vi "Task_03.vi"() -> ()   [LabVIEW 2018]
uses:
  Histogram.ctl
  Stat_cluster.ctl
  <vilib>/Utility/file.llb/Write Delimited Spreadsheet (DBL).vi
panel:
  out "File write error":errorcluster
  out "Histogramm 2":T1
  out "Stats 2":T2
  out "Stats":T2
  out "Histogramm":T1
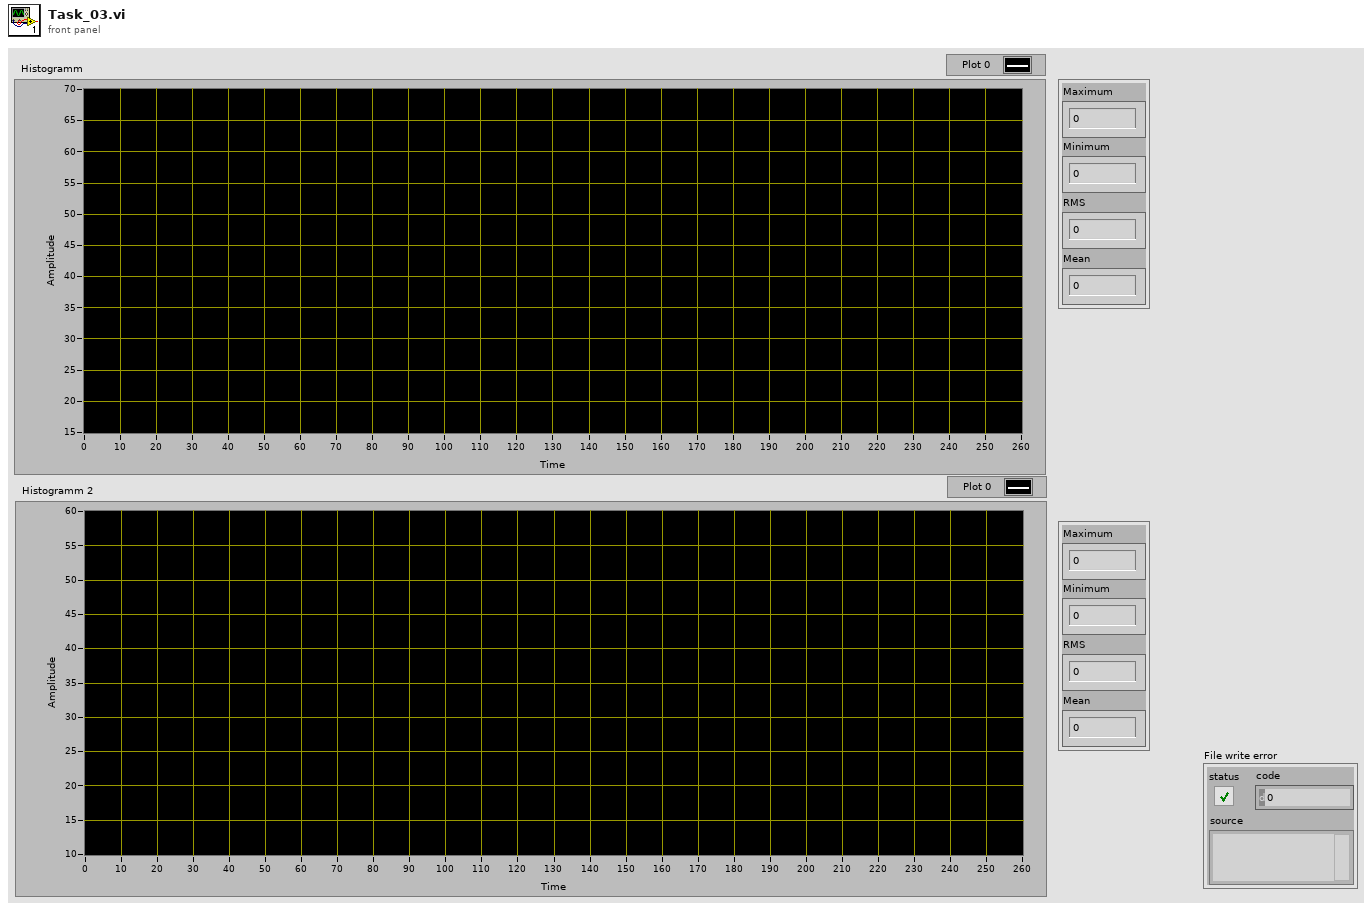
[diagram p1: front panel]
types:
  T1 = typedef "Histogram.ctl" = cluster{"X Values":dbl[], "Histogram: h(x)":i32[]}
  T2 = typedef "Stat_cluster.ctl" = cluster{"Maximum":dbl, "Minimum":dbl, "RMS":dbl, "Mean":dbl}
  T3 = cluster{"Numeric Control":u8, "Numeric Control":u8, "rms value":dbl, "mean":dbl}
  T4 = cluster{"X Values":dbl[], "Histogram: h(x)":i32[]}
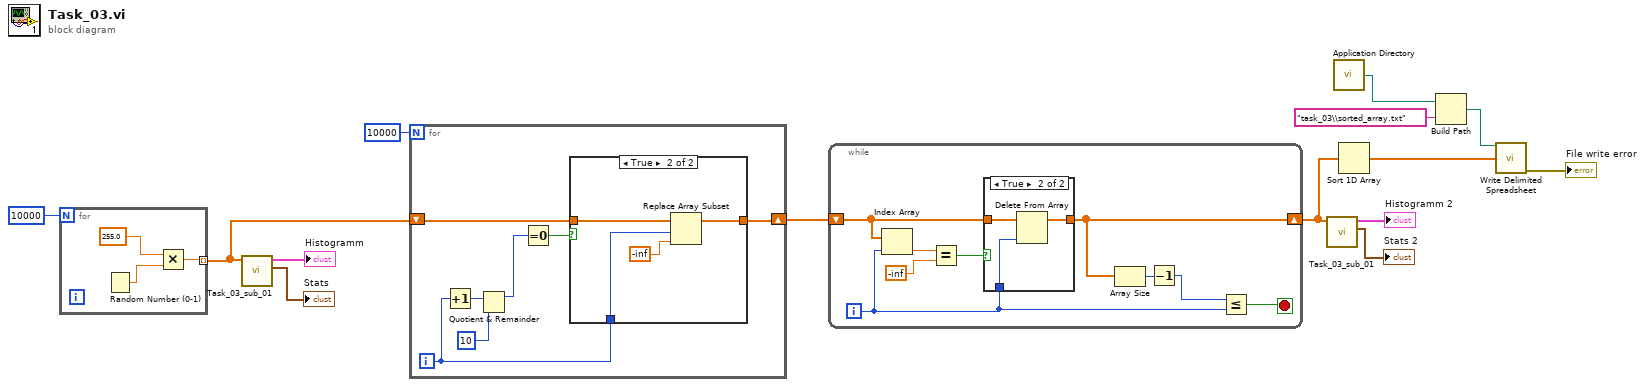
[diagram p0: block diagram]
diagram:
  n1 = for {
    N: 10000 -> [_]
    tunnel: [w15] -> w10 mode=indexing
    n2 = Random Number (0-1)() -> (number: 0 to 1=w16:dbl)
    n3 = Multiply(x=255.0, y=w16) -> (x*y=w15:dbl)
  }
  n4 = call "Task_03_sub_01.vi"("Array"=w10) -> ("Stat_Cluster"=→"Stats":T3, "Histogram Graph"=→"Histogramm":T4)  [unwired: 9 in]
  n5 = for {
    N: 10000 -> [_]
    shift-right: [w19] -> w9
    shift-left: w10 -> [w20]
    i -> [w21]
    n6 = Increment(x=w21) -> (x+1=w24:i32)
    n7 = Quotient & Remainder(x=w24, y=10) -> (x-y*floor(x/y)=w18:i32)  [unwired: 1 out]
    n8 = Equal To 0?(x=w18) -> (x = 0?=w22:bool)
    n9 = case shown="True" w22 {
      tunnel: w21 -> [_ w28]
      tunnel: w20 -> [w25 w29]
      tunnel: [w25 w27] -> w19
      frame False {
      }
      frame True {
        n10 = Replace Array Subset(array=w29, new element=-inf, index=w28) -> (w27:dbl[])
      }
    }
  }
  n11 = while {
    shift-right: [w35] -> w6
    shift-left: w9 -> [w37]
    i -> [w32]
    stop <- w31 stop-if-true
    n12 = Index Array(array=w37, index=w32) -> (element=w38:dbl)
    n13 = Equal?(x=w38, y=-inf) -> (x = y?=w36:bool)
    n14 = case shown="True" w36 {
      tunnel: w37 -> [w39 w42]
      tunnel: w32 -> [_ w41]
      tunnel: [w39 w40] -> w35
      frame False {
      }
      frame True {
        n15 = Delete From Array(array=w42, index=w41) -> (array with subset deleted=w40:dbl[])  [unwired: 1 in, 1 out]
      }
    }
    n16 = Array Size(array=w35) -> (size(s)=w34:i32)
    n17 = Decrement(x=w34) -> (x-1=w33:i32)
    n18 = Less Or Equal?(x=w33, y=w32) -> (x <= y?=w31:bool)
  }
  n19 = call "Task_03_sub_01.vi"("Array"=w6) -> ("Stat_Cluster"=→"Stats 2":T3, "Histogram Graph"=→"Histogramm 2":T4)  [unwired: 9 in]
  n20 = call <vilib>:"Application Directory.vi"() -> ("Application Directory"=w1:path)
  n21 = Sort 1D Array(array=w6) -> (sorted array=w5:dbl[])
  n22 = Build Path(base path=w1, name or relative path="task_03\\sorted_array.txt") -> (appended path=w3:path)
  n23 = call-poly <vilib>:"Write Delimited Spreadsheet.vi"("file path (dialog if empty)"=w3, "1D data"=w5) -> ("error out"=→"File write error":errorcluster)  [unwired: 12 in, 1 out]
